vi "Extract_to_spreadsheet.vi"() -> ()   [LabVIEW 2019]
panel:
  in  "Folder out":path
  in  "Output file name":string
  in  "Samples to average":i32=10000
  in  "Samples per freq calc":i32=10000
  in  "Folder in":path
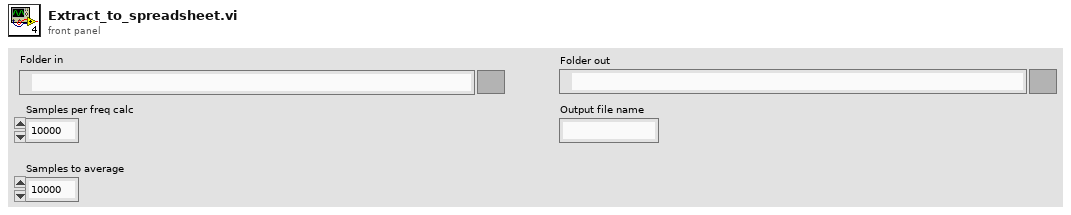
[diagram p1: front panel]
types:
  T1 = enum16{"open", "replace", "create", "open or create", "replace or create", "replace or create with confirmation"}
  T2 = enum16{"open", "open or create", "create or replace", "create", "open (read-only)"}
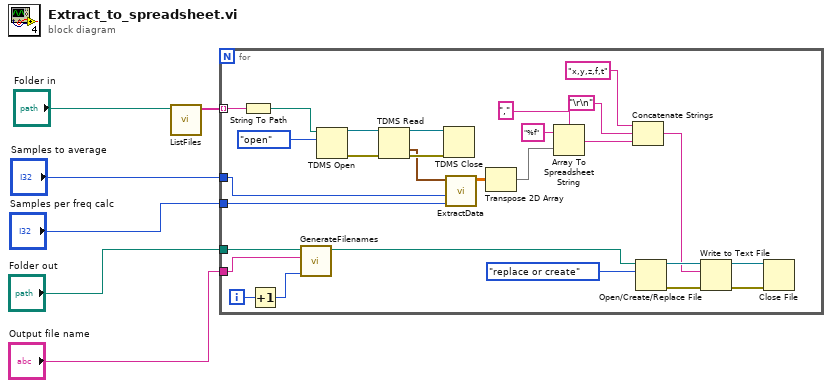
[diagram p0: block diagram]
diagram:
  n1 = call "ListFiles.vi"("Folder"="Folder in") -> ("TDMS"=w5:string[])  [unwired: 10 in]
  n2 = for {
    tunnel: "Samples per freq calc" -> [w28]
    tunnel: w5 -> [w22] mode=indexing
    tunnel: "Samples to average" -> [w21]
    tunnel: "Folder out" -> [w16]
    tunnel: "Output file name" -> [w13]
    i -> [w15]
    n3 = String To Path(string=w22) -> (path=w20:path)
    n4 = Increment(x=w15) -> (x+1=w14:i32)
    n5 = call "GenerateFilenames.vi"("file number"=w14, "filename"=w13, "Path"=w16) -> ("Filepath"=w12:path)  [unwired: 8 in]
    n6 = TDMS Open(10:T2."open" ("operation (0:open)"), 11:w20) -> (0:w32:errorcluster, 3:w33:refnum<k34>)  [unwired: 5 in]
    n7 = TDMS Read(0:w33, 11:w32) -> (4:w31:refnum<k34>, 10:w29:waveform(dbl)[], 15:w30:errorcluster)  [unwired: 6 in, 3 out]
    n8 = TDMS Close(8:w30, 11:w31) -> ()  [unwired: 2 out]
    n9 = call "ExtractData.vi"("Samples per freq calc"=w28, "Samples to average"=w21, "Data input"=w29) -> ("Data array"=w19:dbl[][])  [unwired: 8 in]
    n10 = Transpose 2D Array(2D array=w19) -> (transposed array=w17:dbl[][])
    n11 = Array To Spreadsheet String(delimiter (Tab)=",", array=w17, 3:"%f" ("format string")) -> (spreadsheet string=w10:string)
    n12 = Concatenate Strings("x,y,z,f,t", "\r\n", w10) -> (w11:string)
    n13 = Open/Create/Replace File(file path (use dialog)=w12, operation (0:open)=T1."replace or create") -> (refnum out=w25:refnum<file>, error out=w24:errorcluster)  [unwired: 4 in, 1 out]
    n14 = Write to Text File(file (use dialog)=w25, text=w11, error in=w24) -> (refnum out=w27:refnum<file>, error out=w26:errorcluster)  [unwired: 1 in, 1 out]
    n15 = Close File(refnum=w27, error in=w26) -> ()  [unwired: 2 out]
  }
